vi "MSScript_Format_AcqSig.vi"(9 "ValueArray":string[](array[string]), 10 "TagArray":string[](array[string]), 11 "MSScript in":refnum<class "MSScript.lvclass">) -> (0 "ValueErrorArray":bool[](array[boolean]), 1 "TagErrorArray":bool[](array[boolean]), 2 "ParamErrorArray":bool[](array[boolean]), 3 "Data":variant, 4 "#ofParamError":bool)   [LabVIEW 2018, in "MSScript.lvclass"]
uses:
  MSScript.lvclass
  Ctl/MSEditorParam acqSig.ctl
  MSScript_Transform_Extended.vi
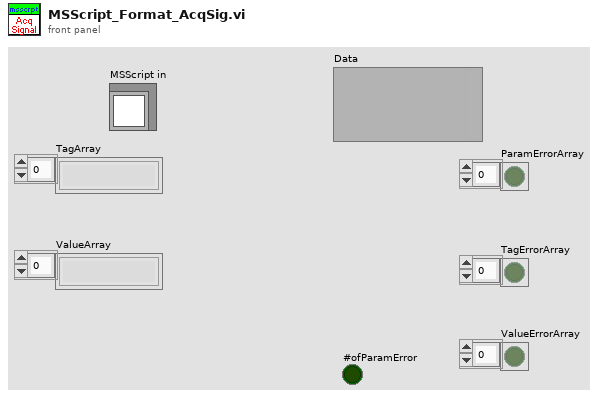
[diagram p1: front panel]
types:
  T1 = typedef "MSEditorParam acqSig.ctl" = cluster{"time ":dbl}
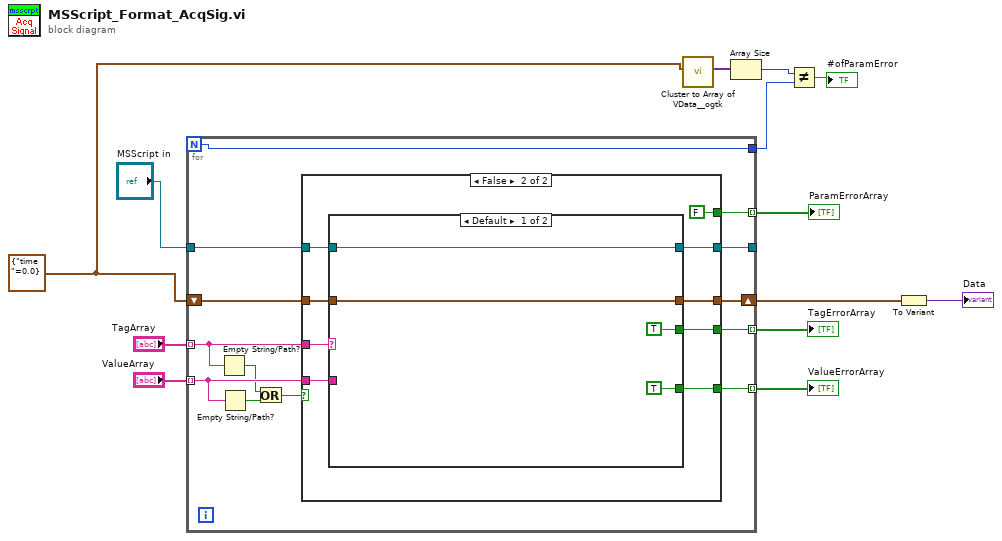
[diagram p0: block diagram]
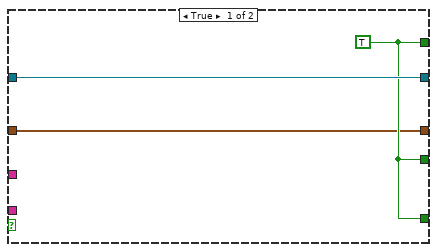
[diagram p2: hidden frame]
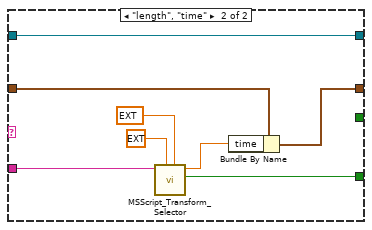
[diagram p3: hidden frame]
diagram:
  w3 = T1 {"time "=0.0} ("ParamValueType")
  n1 = for {
    N -> [w14]
    tunnel: "TagArray" -> [w22] mode=indexing
    tunnel: "ValueArray" -> [w21] mode=indexing
    tunnel: [w26] -> w11 mode=indexing
    tunnel: "MSScript in" -> [w25]
    tunnel: [w24] -> w10 mode=indexing
    tunnel: [w23] -> _
    tunnel: [w17] -> w9 mode=indexing
    shift-right: [w15] -> w2
    shift-left: w3 -> [w16]
    tunnel: [w14] -> w4
    n2 = Empty String/Path?(string/path=w22) -> (empty?=w19:bool)
    n3 = Empty String/Path?(string/path=w21) -> (empty?=w20:bool)
    n4 = Or(x=w19, y=w20) -> (x .or. y?=w18:bool)
    n5 = case shown="False" w18 {
      tunnel: [w28 w31] -> w26
      tunnel: w25 -> [w29 w37]
      tunnel: [w28 w30] -> w24
      tunnel: [w29 w33] -> w23
      tunnel: w22 -> [_ w35]
      tunnel: w21 -> [_ w34]
      tunnel: [w28 FALSE] -> w17
      tunnel: w16 -> [w27 w36]
      tunnel: [w27 w32] -> w15
      frame True {
        w28 = TRUE
      }
      frame False {
        n6 = case shown="Default" w35 {
          tunnel: [TRUE _] -> w31
          tunnel: w37 -> [w40 w48]
          tunnel: w34 -> [_ w49]
          tunnel: [TRUE ("Value Error?") w50] -> w30
          tunnel: [w40 w48] -> w33
          tunnel: w36 -> [w39 w46]
          tunnel: [w39 w45] -> w32
          frame Default {
          }
          frame "length", "time" {
            n7 = call-poly "MSScript_Transform_Selector.vi"("upper limit (Inf)"=ext 300.0, "lower limit (-Inf)"=ext 0.0, "Check_Str"=w49) -> ("Value Error?"=w50:bool, "Value Output"=w47:ext)  [unwired: 6 in, 1 out]
            n8 = Bundle By Name(cluster=w46, "time"=w47) -> (w45:T1)
          }
        }
      }
    }
  }
  "TagErrorArray" <- w11
  "ValueErrorArray" <- w10
  "ParamErrorArray" <- w9
  n9 = call <userlib>:"Cluster to Array of VData__ogtk.vi"("Cluster"=w3) -> ("Array of VData"=w7:variant[])  [unwired: 9 in, 1 out]
  n10 = Array Size(array=w7) -> (size(s)=w6:i32)
  n11 = Not Equal?(x=w6, y=w4) -> (x != y?=→"#ofParamError":bool)
  n12 = To Variant(anything=w2) -> (Variant=→"Data":variant)
